vi "add.vi"(8 "error in (no error)":errorcluster, 9 "constant":sgl, 10 "addend":refnum<class "Image.lvclass">=refnum, 11 "Image in":refnum<class "Image.lvclass">=refnum) -> (0 "error out":errorcluster, 3 "Image out":refnum<class "Image.lvclass">)   [LabVIEW 2010, in "Image.lvclass"]
uses:
  helioscan/bricks/classes/Image/Image.lvclass
  helioscan/bricks/classes/Image/storage_mode.ctl
panel:
  in  "Number of samples per revolution":i16=1000
  in  "Length 2b (um)":dbl=30.0
  in  "Length 2a (um)":dbl=50.0
  in  "Phase shift (fraction of pi)":dbl
  in  "Frequency ration b":dbl=1.0
  in  "Frequency ratio a":dbl=1.0
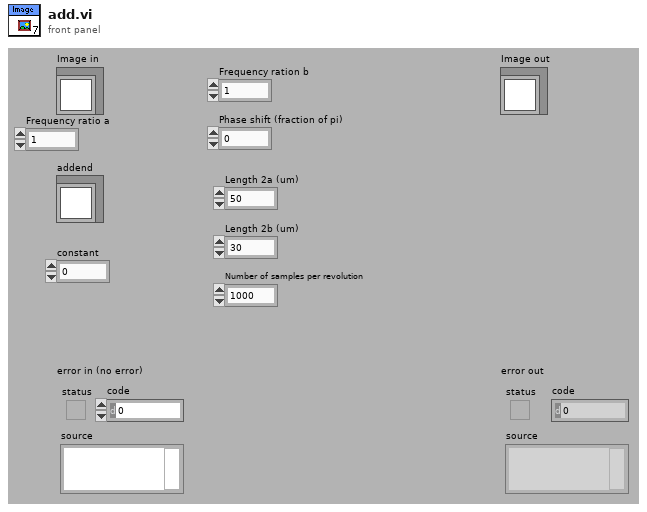
[diagram p1: front panel]
types:
  T1 = typedef "Image.lvclass/storage_mode.ctl" = enum16{"RAM", "disk"}
  T2 = typedef "IMAQ Image.ctl" = refnum<image>
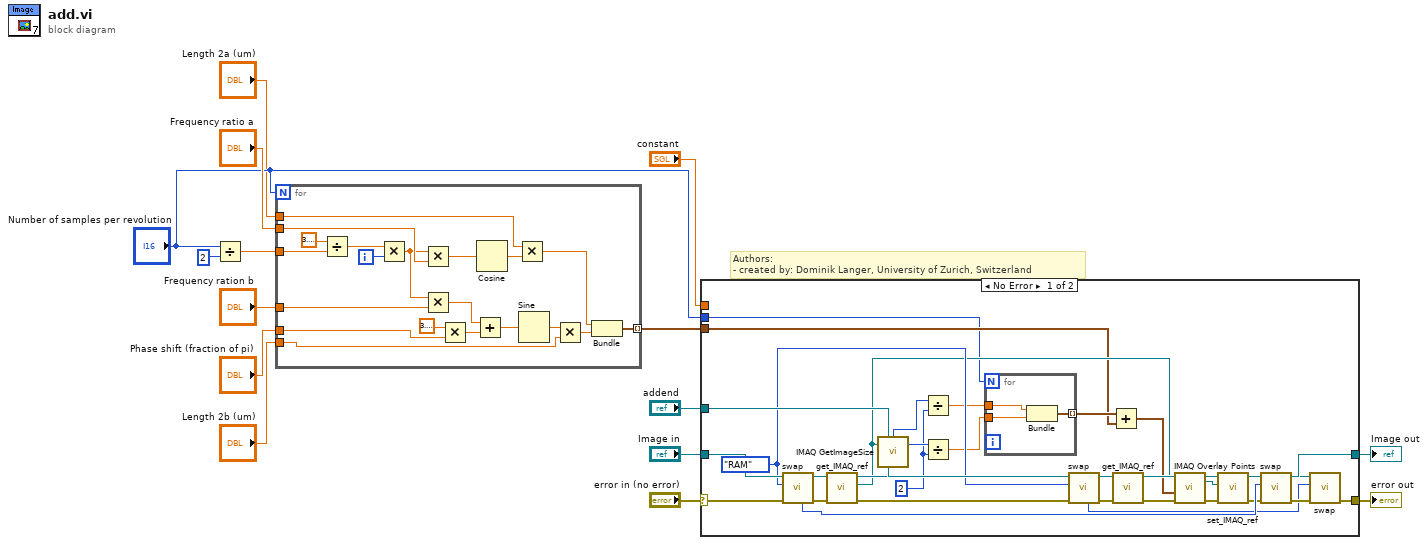
[diagram p0: block diagram]
diagram:
  # "Authors: \n- created by: Dominik Langer, University of Zurich, Switzerland"
  n1 = Divide(x="Number of samples per revolution", y=2) -> (x/y=w8:dbl)
  n2 = for {
    N: "Number of samples per revolution" -> [_]
    tunnel: [w34] -> w3 mode=indexing
    tunnel: "Length 2a (um)" -> [w30]
    tunnel: "Length 2b (um)" -> [w27]
    tunnel: "Phase shift (fraction of pi)" -> [w23]
    tunnel: w8 -> [w26]
    tunnel: "Frequency ratio a" -> [w21]
    tunnel: "Frequency ration b" -> [w19]
    i -> [w32]
    n3 = Divide(x=3.141592653589793, y=w26) -> (x/y=w35:dbl)
    n4 = Multiply(x=w35, y=w32) -> (x*y=w20:dbl)
    n5 = Multiply(x=w20, y=w21) -> (x*y=w22:dbl)
    n6 = Multiply(x=w20, y=w19) -> (x*y=w18:dbl)
    n7 = Multiply(x=3.141592653589793, y=w23) -> (x*y=w25:dbl)
    n8 = Add(x=w18, y=w25) -> (x+y=w31:dbl)
    n9 = Cosine(x=w22) -> (cos(x)=w29:dbl)
    n10 = Multiply(x=w30, y=w29) -> (x*y=w16:dbl)
    n11 = Sine(x=w31) -> (sin(x)=w28:dbl)
    n12 = Multiply(x=w28, y=w27) -> (x*y=w17:dbl)
    n13 = Bundle(w16, w17) -> (w34:cluster{dbl, dbl})  [unwired: 1 out]
  }
  n14 = case shown="No Error" "error in (no error)" {
    selector: "error in (no error)" -> [w62 w71]
    tunnel: [w51 w71] -> w14
    tunnel: [w54 w70] -> w12
    tunnel: "Image in" -> [w59 w70]
    tunnel: "addend" -> [w66 _]
    tunnel: "constant" -> [_ _]
    tunnel: w3 -> [w37 _]
    tunnel: "Number of samples per revolution" -> [w36 _]
    frame No Error {
      w57 = storage_mode."RAM" ("storage type target")
      w42 = 2
      n15 = call-dynamic "swap.vi"("error in (no error)"=w62, "storage type target"=w57, "Image in"=w59) -> ("error out"=w63:errorcluster, "Image out"=w60:refnum<class "Image.lvclass">, "previous storage mode"=w56:T1)  [unwired: 6 out]
      n16 = call-dynamic "get_IMAQ_ref.vi"("error in (no error)"=w63, "Image.lvclass in"=w60) -> ("error out"=w61:errorcluster, "Image"=w40:T2, "Image.lvclass out"=w58:refnum<class "Image.lvclass">)  [unwired: 7 out]
      n17 = call "IMAQ GetImageSize"("Image"=w40) -> ("Y Resolution"=w43:i32, "X Resolution"=w41:i32)  [unwired: 1 in, 3 out]
      n18 = Divide(x=w41, y=w42) -> (x/y=w44:dbl)
      n19 = Divide(x=w43, y=w42) -> (x/y=w45:dbl)
      n20 = for {
        N: w36 -> [_]
        tunnel: w44 -> [w69]
        tunnel: w45 -> [w68]
        tunnel: [w67] -> w38 mode=indexing
        n21 = Bundle(w69, w68) -> (w67:cluster{dbl, dbl})  [unwired: 1 out]
      }
      n22 = call-dynamic "swap.vi"("error in (no error)"=w61, "storage type target"=w57, "Image in"=w66) -> ("error out"=w65:errorcluster, "Image out"=w64:refnum<class "Image.lvclass">, "previous storage mode"=w49:T1)  [unwired: 6 out]
      n23 = Add(x=w38, y=w37) -> (x+y=w39:cluster{dbl, dbl}[])
      n24 = call-dynamic "get_IMAQ_ref.vi"("error in (no error)"=w65, "Image.lvclass in"=w64) -> ("error out"=w46:errorcluster, "Image.lvclass out"=w50:refnum<class "Image.lvclass">)  [unwired: 8 out]
      n25 = call "IMAQ Overlay Points"("error in (no error)"=w46, "Array of Points"=w39, "Image"=w40) -> ("error out"=w47:errorcluster, "Image Out"=w48:T2)  [unwired: 3 in, 4 out]
      n26 = call-dynamic "set_IMAQ_ref.vi"("error in (no error)"=w47, "Image"=w48, "Image.lvclass in"=w58) -> ("error out"=w53:errorcluster, "Image.lvclass out"=w55:refnum<class "Image.lvclass">)  [unwired: 7 out]
      n27 = call-dynamic "swap.vi"("error in (no error)"=w53, "storage type target"=w56, "Image in"=w55) -> ("error out"=w52:errorcluster, "Image out"=w54:refnum<class "Image.lvclass">)  [unwired: 7 out]
      n28 = call-dynamic "swap.vi"("error in (no error)"=w52, "storage type target"=w49, "Image in"=w50) -> ("error out"=w51:errorcluster)  [unwired: 8 out]
    }
    frame Error {
    }
  }
  "error out" <- w14
  "Image out" <- w12
